vi "PathPlanner_Cmd_AutoInitFromJsonData.vi"(8 "Cmd Index":i32, 10 "JSON String":string, 11 "In Command Data":T2) -> (0 "error out":errorcluster, 3 "out Command Data":T2)   [LabVIEW 2019, in "PathPlanner24.lvlib"]
doc: "Internal function to parse JSON data for Event Markers. This is data that is different for each different type of Event Marker command.\n\nNotes:\n--------\nCurrently the only type of commands that can be issued are Boolean commands. The value is forced to TRUE when the command is issued.\n\nThe following table lists the actions performed for different types of commands:\n - Unknown - nothing - not supported.\n - Wait - nothing - not supported\n - Named - Issue boolean command with TRUE value using the \"name\" as the command name.\n - Path - nothing - not supported\n - Sequential, Parallel, Race, Deadline - Issue boolean command with TRUE value for each of the commands contained in the \"commands\" array. The value for \"name\" is used as the command name."
uses:
  PathPlanner24.lvlib
  ENum/PathPlanner_CommandUtil_Type_ENUM.ctl
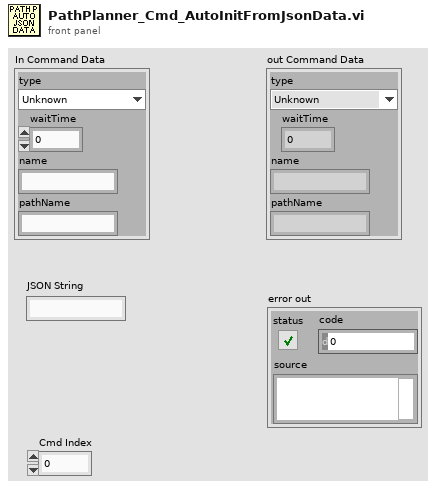
[diagram p1: front panel]
types:
  T1 = typedef "PathPlanner24.lvlib/PathPlanner_CommandUtil_Type_ENUM.ctl" = enum16{"Unknown", "Wait", "Named", "Path", "Sequential", "Parallel", "Race", "Deadline", "PointTowardsZoneEnter", "PointTowardsZoneExit", "TriggerEventStart", "TriggerEventStop", "TriggerEventOneshot"}
  T2 = cluster{"type":T1, "waitTime":dbl, "name":string, "pathName":string}
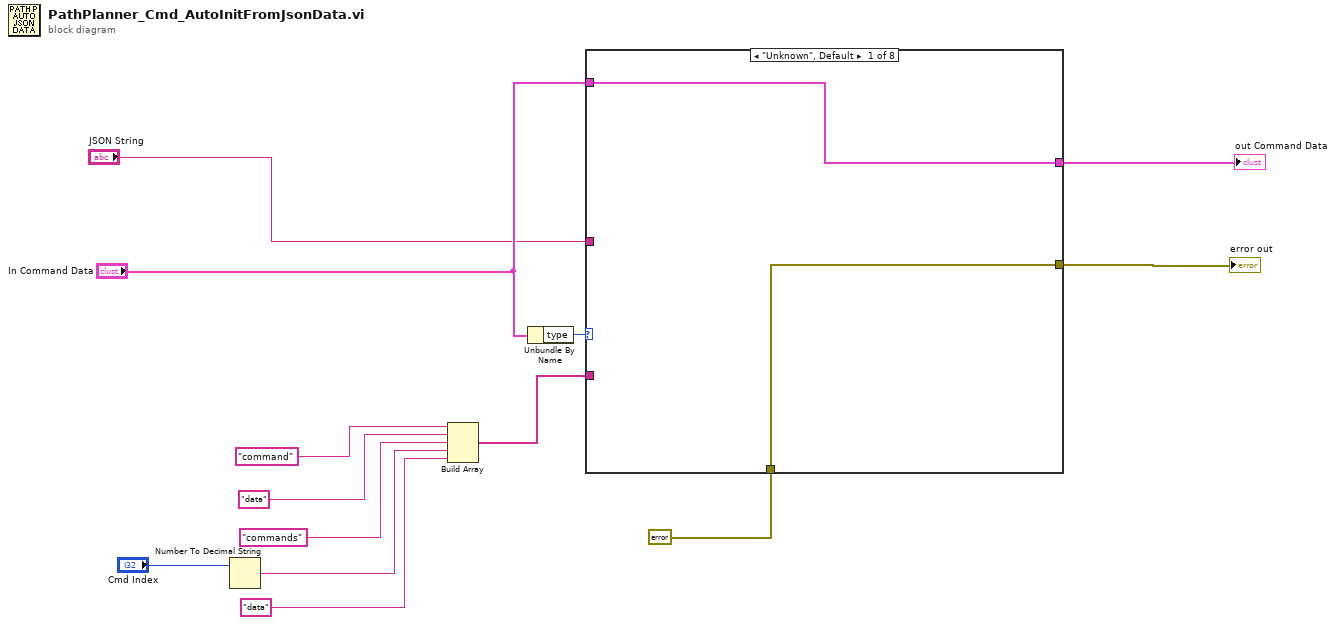
[diagram p0: block diagram]
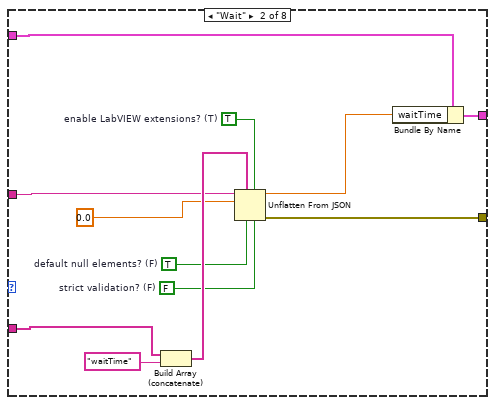
[diagram p2: hidden frame]
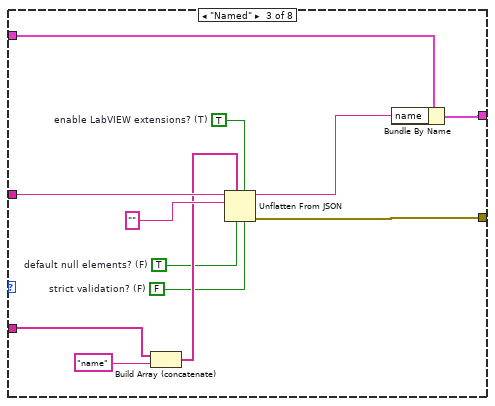
[diagram p3: hidden frame]
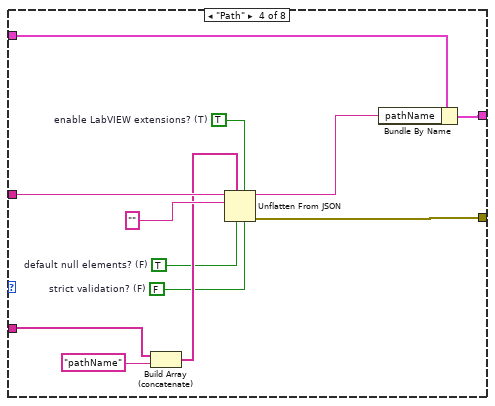
[diagram p4: hidden frame]
diagram:
  n1 = Number To Decimal String(number="Cmd Index") -> (decimal integer string=w8:string)  [unwired: 1 in]
  n2 = Build Array("command", "data", "commands", w8, "data") -> (w4:string[])
  n3 = Unbundle By Name("In Command Data") -> ("type"=w13:T1)
  n4 = case shown="\"Unknown\", Default" w13 {
    tunnel: "In Command Data" -> [w15 w20 w30 w42 w53 w55 w57 w59]
    tunnel: [w15 w17 w31 w43 w53 w55 w57 w59] -> w5
    tunnel: w4 -> [_ w21 w39 w51 _ _ _ _]
    tunnel: "JSON String" -> [_ w19 w37 w49 _ _ _ _]
    tunnel: [w14 w16 w28 w40 w52 w54 w56 w58] -> w2
    tunnel: errorcluster {"status"=FALSE, "code"=0, "source"=""} ("error out") -> [w14 _ _ _ w52 w54 w56 w58]
    frame "Unknown", Default {
    }
    frame "Wait" {
      w23 = FALSE  # strict validation? (F)
      w24 = TRUE  # default null elements? (F)
      w25 = TRUE  # enable LabVIEW extensions? (T)
      n5 = Build Array (concatenate)(w21, "waitTime") -> (w26:string[])
      n6 = Unflatten From JSON(path=w26, enable LabVIEW extensions? (T)=w25, JSON string=w19, type and defaults=0.0, default null elements? (F)=w24, strict validation? (F)=w23) -> (value=w22:dbl, error out=w16:errorcluster)  [unwired: 1 in]
      n7 = Bundle By Name(cluster=w20, "waitTime"=w22) -> (w17:T2)
    }
    frame "Named" {
      w32 = FALSE  # strict validation? (F)
      w33 = TRUE  # default null elements? (F)
      w34 = TRUE  # enable LabVIEW extensions? (T)
      n8 = Build Array (concatenate)(w39, "name") -> (w35:string[])
      n9 = Unflatten From JSON(path=w35, enable LabVIEW extensions? (T)=w34, JSON string=w37, type and defaults="", default null elements? (F)=w33, strict validation? (F)=w32) -> (value=w29:string, error out=w28:errorcluster)  [unwired: 1 in]
      n10 = Bundle By Name(cluster=w30, "name"=w29) -> (w31:T2)
    }
    frame "Path" {
      w44 = FALSE  # strict validation? (F)
      w45 = TRUE  # default null elements? (F)
      w46 = TRUE  # enable LabVIEW extensions? (T)
      n11 = Build Array (concatenate)(w51, "pathName") -> (w47:string[])
      n12 = Unflatten From JSON(path=w47, enable LabVIEW extensions? (T)=w46, JSON string=w49, type and defaults="", default null elements? (F)=w45, strict validation? (F)=w44) -> (value=w41:string, error out=w40:errorcluster)  [unwired: 1 in]
      n13 = Bundle By Name(cluster=w42, "pathName"=w41) -> (w43:T2)
    }
    frame "Sequential" {
      # "shouldn't get this."
    }
    frame "Parallel" {
      # "Shouldn't get this."
    }
    frame "Race" {
      # "Shouldn't get this."
    }
    frame "Deadline" {
      # "Shouldn't get this."
    }
  }
  "out Command Data" <- w5
  "error out" <- w2
